vi "New TDMS Log File.vi"(4 "File Properties":T2[](array[typedef]), 6 "File Description":string, 7 "Apply Root Properties to Groups":bool, 8 "error in (no error)":errorcluster, 9 "Channel Groups":T4[](array[typedef]), 10 "File Conflict Operation":T3, 11 "Log File Path":path) -> (0 "error out":errorcluster, 3 "TDMSLogFile Ref":T1)   [LabVIEW 2020, in "NI_VS Data Logging API.lvlib"]
uses:
  <vilib>/NI VeriStand/Execution/DataLogging/NI_VS Data Logging API.lvlib
  <vilib>/NI VeriStand/Execution/DataLogging/TDMS Channel Group.ctl
  <vilib>/NI VeriStand/Execution/DataLogging/TDMS Property.ctl
  <vilib>/NI VeriStand/Execution/DataLogging/TDMS Channel.ctl
  <vilib>/NI VeriStand/Execution/DataLogging/Time Channel Options.ctl
  <vilib>/NI VeriStand/Execution/DataLogging/File Conflict Operation.ctl
  <vilib>/NI VeriStand/Execution/DataLogging/TdmsLogFile Ref.ctl
  NationalInstruments.VeriStand.ClientAPI
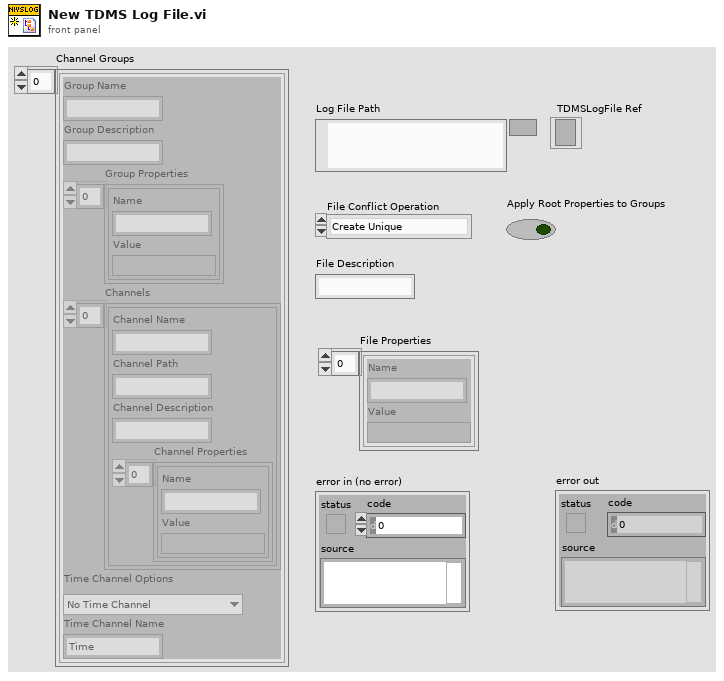
[diagram p1: front panel]
types:
  T1 = typedef "NI_VS Data Logging API.lvlib/TdmsLogFile Ref.ctl" = refnum<k24>
  T2 = typedef "NI_VS Data Logging API.lvlib/TDMS Property.ctl" = cluster{"Name":string, "Value":variant}
  T3 = typedef "NI_VS Data Logging API.lvlib/File Conflict Operation.ctl" = enum16{"Create Unique", "Append to Existing", "Overwrite"}
  T4 = typedef "NI_VS Data Logging API.lvlib/TDMS Channel Group.ctl" = cluster{"Group Name":string, "Group Description":string, "Group Properties":T2[], "Channels":T5[], "Time Channel Options":T6, "Time Channel Name":string}
  T5 = typedef "NI_VS Data Logging API.lvlib/TDMS Channel.ctl" = cluster{"Channel Name":string, "Channel Path":string, "Channel Description":string, "Channel Properties":T2[]}
  T6 = typedef "NI_VS Data Logging API.lvlib/Time Channel Options.ctl" = enum16{"No Time Channel", "Absolute Time", "System Time", "System Time - Microseconds", "Absolute Time as Double", "Relative To First Start Trigger", "Relative To Session Start"}
  T7 = typedef "NI_VS Data Logging API.lvlib/TdmsProperty Ref.ctl" = refnum<k24>
  T8 = typedef "NI_VS Data Logging API.lvlib/TdmsChannelGroup Ref.ctl" = refnum<k24>
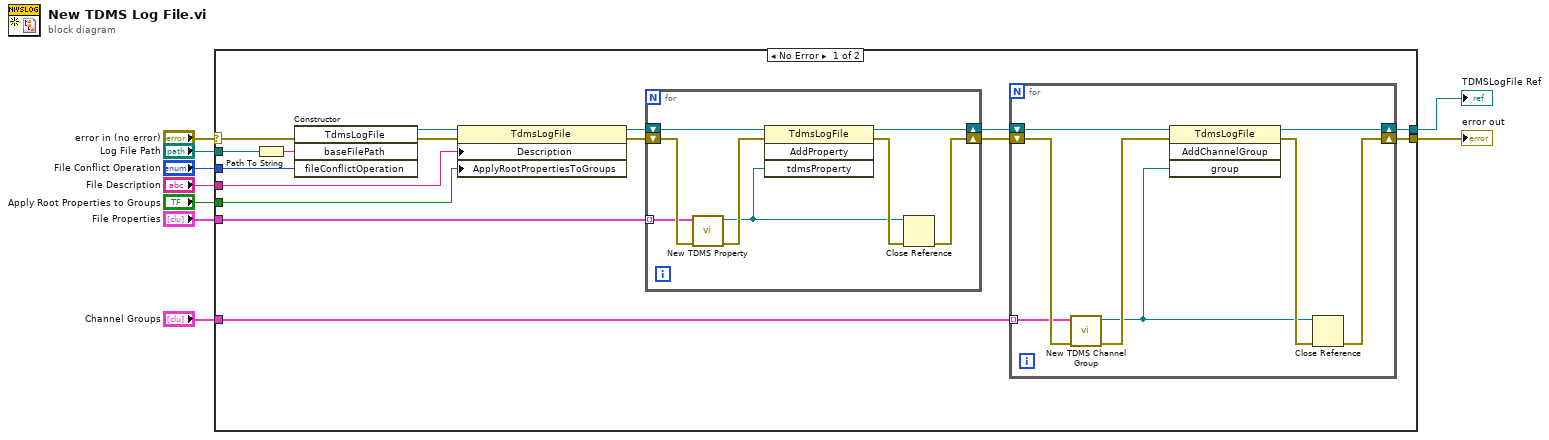
[diagram p0: block diagram]
diagram:
  n1 = case shown="No Error" "error in (no error)" {
    selector: "error in (no error)" -> [w25 w42]
    tunnel: [w12 w42] -> w8
    tunnel: "Log File Path" -> [w24 _]
    tunnel: "File Conflict Operation" -> [w22 _]
    tunnel: "File Description" -> [w19 _]
    tunnel: "File Properties" -> [w18 _]
    tunnel: "Channel Groups" -> [w14 _]
    tunnel: [w11 _] -> w2
    tunnel: "Apply Root Properties to Groups" -> [w10 _]
    frame No Error {
      n2 = Path To String(path=w24) -> (string=w23:string)
      n3 = constructor class="TdmsLogFile"(error in=w25, "baseFilePath"=w23, "fileConflictOperation"=w22) -> (reference out=w21:refnum<k24>, error out=w20:errorcluster)  [unwired: 2 in, 3 out]
      n4 = property class="TdmsLogFile"(reference=w21, error in=w20, "Description"=w19, "ApplyRootPropertiesToGroups"=w10) -> (reference out=w17:refnum<k24>, error out=w16:errorcluster)
      n5 = for {
        tunnel: w18 -> [w37] mode=indexing
        shift-right: [w38] -> w15
        shift-left: w17 -> [w39]
        shift-right: [w34] -> w13
        shift-left: w16 -> [w40]
        n6 = call <vilib>:"New TDMS Property.vi"("error in (no error)"=w40, "TDMS Property"=w37) -> ("error out"=w41:errorcluster, "TDMSProperty Ref"=w35:T7)  [unwired: 8 in]
        n7 = invoke class="TdmsLogFile" method="AddProperty"(reference=w39, error in=w41, "tdmsProperty"=w35) -> (reference out=w38:refnum<k24>, error out=w36:errorcluster)  [unwired: 1 in, 2 out]
        n8 = Close Reference(reference=w35, error in (no error)=w36) -> (error out=w34:errorcluster)
      }
      n9 = for {
        tunnel: w14 -> [w29] mode=indexing
        shift-right: [w27] -> w11
        shift-left: w15 -> [w28]
        shift-right: [w31] -> w12
        shift-left: w13 -> [w33]
        n10 = call <vilib>:"New TDMS Channel Group.vi"("error in (no error)"=w33, "TDMS Channel Group"=w29) -> ("error out"=w30:errorcluster, "TdmsChannelGroup Ref"=w26:T8)  [unwired: 8 in]
        n11 = invoke class="TdmsLogFile" method="AddChannelGroup"(reference=w28, error in=w30, "group"=w26) -> (reference out=w27:refnum<k24>, error out=w32:errorcluster)  [unwired: 1 in, 2 out]
        n12 = Close Reference(reference=w26, error in (no error)=w32) -> (error out=w31:errorcluster)
      }
    }
    frame Error {
    }
  }
  "error out" <- w8
  "TDMSLogFile Ref" <- w2
